vi "NPC3SG Close.vi"(4 "Drive Visa Name":refnum<visa-resource-name>) -> ()   [LabVIEW 2010]
uses:
  drivers/Newport NPC3SG/SubNPC3SG.llb/device variables.vi
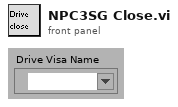
[diagram p1: front panel]
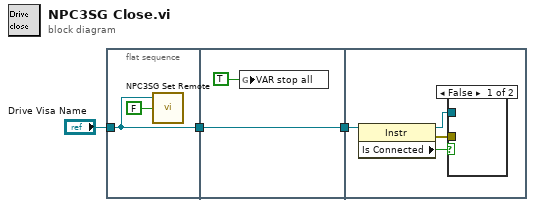
[diagram p0: block diagram]
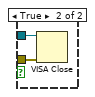
[diagram p2: hidden frame]
diagram:
  n1 = flat-sequence {
    tunnel: "Drive Visa Name" -> [w4]
    tunnel: [w4] -> w1
    tunnel: [w6] -> w2
    tunnel: w1 -> [w6]
    tunnel: w2 -> [w8]
    frame #0 {
      n2 = call "NPC3SG Set Remote.vi"("Remote?"=FALSE, "Drive Visa Name"=w4) -> ()  [unwired: 1 in, 2 out]
    }
    frame #1 {
      n3 = global write "device variables.vi" "VAR stop all"(TRUE ("VAR stop all")) -> ()
    }
    frame #2 {
      n4 = property class="Instr"(reference=w8) -> (reference out=w10:refnum<visa-resource-name>, error out=w11:errorcluster, "Is Connected"=w9:bool)  [unwired: 1 in]
      n5 = case shown="False" w9 {
        tunnel: w10 -> [_ w13]
        tunnel: w11 -> [_ w12]
        frame False {
        }
        frame True {
          n6 = VISA Close(VISA resource name=w13, error in (no error)=w12) -> ()  [unwired: 1 out]
        }
      }
    }
  }
